vi "Replace Default with Tag.vi"(5 "instance id":string, 7 "engine configuration in":refnum<class "engine configuration.lvclass">, 9 "Channel Index":i32, 10 "Channel":refnum<class "TBM channel.lvclass">, 11 "Array in":string[](array[string])) -> (3 "Array out":string[](array[string]))   [LabVIEW 2015, in "PID Module configuration.lvclass"]
uses:
  module/configuration/PID Module configuration.lvclass
  <vilib>/NI/Module Execution Interface/Engine Configuration/engine configuration.lvclass
  <vilib>/NI/Tag Bus Module Framework/channel/TBM channel.lvclass
  <vilib>/NI/Tag Bus/tag/tag descriptor.lvclass/tag descriptor.ctl
  <vilib>/NI/Tag Bus/tag/tag descriptor.lvclass
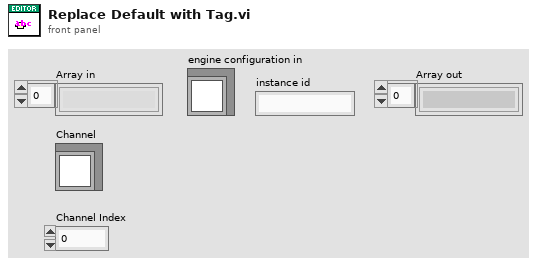
[diagram p1: front panel]
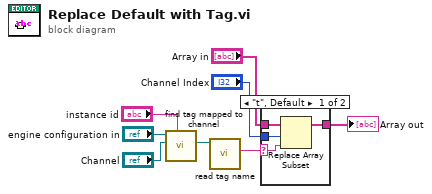
[diagram p0: block diagram]
diagram:
  n1 = call <vilib>:"find tag mapped to channel.vi"("owner"="instance id", "channel"="Channel", "engine configuration in"="engine configuration in") -> ("tag"=w7:refnum<class "tag descriptor.lvclass">)  [unwired: 6 in, 2 out]
  n2 = call <vilib>:"read tag name.vi"("system tag in"=w7) -> ("name"=w4:string)  [unwired: 8 in, 2 out]
  n3 = case shown="\"t\", Default" w4 {
    selector: w4 -> [w12 _]
    tunnel: [w10 w13] -> w3
    tunnel: "Array in" -> [w11 w13]
    tunnel: "Channel Index" -> [w9 _]
    frame "t", Default {
      n4 = Replace Array Subset(array=w11, new element=w12, index=w9) -> (w10:string[])
    }
    frame "" {
    }
  }
  "Array out" <- w3
